vi "launcher.vi"   [LabVIEW 2018, in "launcher.lvlib"]
uses:
  launcher.lvlib
  <vilib>/ActorFramework/Actor/Actor.lvclass
  UI/UI/UI.lvclass
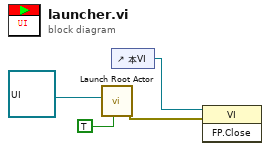
[diagram p0: block diagram]
diagram:
  n1 = call <vilib>:"Launch Root Actor.vi"("Open Actor Core front panel? (F)"=TRUE, "Actor"=refnum<class "UI.lvclass"> refnum ("UI.lvlib:UI.lvclass")) -> ("error out"=w2:errorcluster)  [unwired: 8 in, 1 out]
  n2 = control-ref of="本VI"() -> (w1:refnum<vi>)
  n3 = invoke class="VI" method="FP.Close"(reference=w1, error in=w2) -> ()  [unwired: 1 in, 3 out]
